vi "servo oscillation_rahul 1.vi"() -> ()   [LabVIEW 2012]
uses:
  <vilib>/Motion/FlexMotion/FunctionsVIs/AxisResourceConfig.llb/Enable Axes (8 axes).flx
  <vilib>/Motion/FlexMotion/FunctionsVIs/Trajectory.llb/Load Acceleration/Deceleration.flx
  <vilib>/Motion/FlexMotion/FunctionsVIs/StartStopMotion.llb/Blend Motion (8 axes).flx
  <vilib>/Motion/FlexMotion/FunctionsVIs/StartStopMotion.llb/Start Motion (8 axes).flx
  <vilib>/Motion/FlexMotion/FunctionsVIs/Trajectory.llb/Check Blend Complete Status (8 axes).flx
  <vilib>/Motion/FlexMotion/FunctionsVIs/Trajectory.llb/Check Move Complete Status (8 axes).flx
  <vilib>/Motion/FlexMotion/FunctionsVIs/StartStopMotion.llb/Stop Motion (8 axes).flx
  <vilib>/Analysis/NI_AALBase.lvlib
panel:
  out "Current Position":dbl(slide) scale=-20000.0..20000.0
  in  "STOP":bool
  in  "samples per cycle":dbl=10.0
  in  "no of cycles":dbl=1.0
  in  "amplitude":dbl=15000.0 format="%0.2f"
  in  "RUN":bool
  in  "Acceleration":dbl=100000.0
  in  "Velocity":dbl=10000.0 min=-20000000.0 max=20000000.0
  in  "Board ID":T1=1 min=1 max=32 step=1
  in  "Axis Cluster":T2
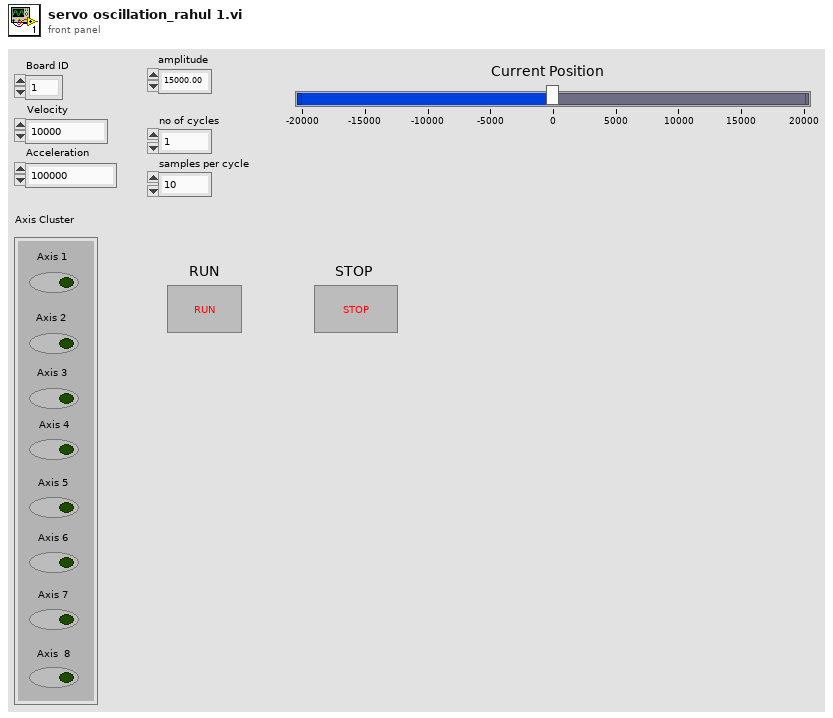
[diagram p1: front panel]
types:
  T1 = typedef "Board Id" = u8
  T2 = cluster{"Axis 1":bool, "Axis 2":bool, "Axis 3":bool, "Axis 4":bool, "Axis 5":bool, "Axis 6":bool, "Axis 7":bool, "Axis  8":bool}
  T3 = enum16{"Absolute Position", "Relative Position", "Velocity", "Relative to Cap Pos", "Modulus Position", "Absolute Contouring", "Relative Contouring"}
  T4 = typedef "Bd Id Out" = u8
  T5 = typedef "Resource Out (Enum).flx" = u16
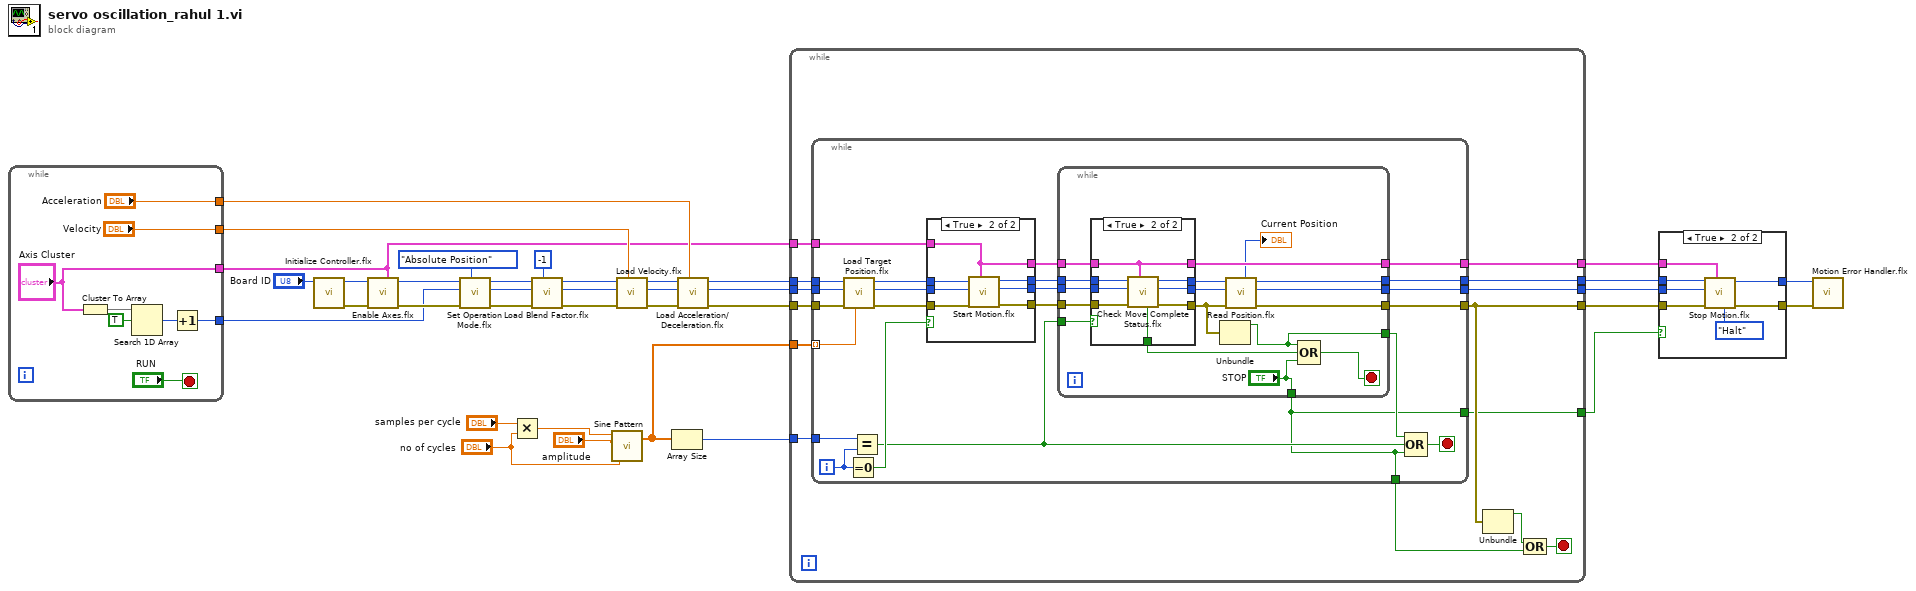
[diagram p0: block diagram]
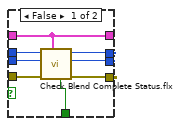
[diagram p2: hidden frame]
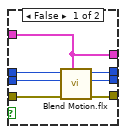
[diagram p3: hidden frame]
diagram:
  n1 = while {
    tunnel: ["Axis Cluster"] -> w14
    tunnel: [w39] -> w20
    tunnel: ["Velocity"] -> w19
    tunnel: ["Acceleration"] -> w18
    stop <- "RUN" stop-if-true
    n2 = Cluster To Array(cluster="Axis Cluster") -> (array=w43:bool[])
    n3 = Search 1D Array(1D array=w43, element=TRUE) -> (index of element=w41:i32)  [unwired: 1 in]
    n4 = Increment(x=w41) -> (x+1=w39:i32)
  }
  n5 = call <vilib>:"Initialize Controller.flx"("Board ID"="Board ID") -> ("error out"=w35:errorcluster, "Bd ID Out"=w36:T4)  [unwired: 7 in]
  n6 = call-poly <vilib>:"Enable Axes.flx"("Axis Bitmap (Disabled)"=w14, "error in (no error)"=w35, "Board ID"=w36) -> ("error out"=w34:errorcluster, "Bd ID Out"=w33:T4)  [unwired: 5 in]
  n7 = call <vilib>:"Set Operation Mode.flx"("Position Mode (Absolute)"=T3."Absolute Position", "error in (no error)"=w34, "Axis or Vector Space"=w20, "Board ID"=w33) -> ("error out"=w26:errorcluster, "Resource Output"=w25:T5, "Bd ID Out"=w27:T4)  [unwired: 2 in]
  n8 = Multiply(x="samples per cycle", y="no of cycles") -> (x*y=w11:dbl)
  n9 = call <vilib>:"Load Blend Factor.flx"("Blend Factor (-1)"=i16 -1, "error in (no error)"=w26, "Axis or Vector Space"=w25, "Board ID"=w27) -> ("error out"=w22:errorcluster, "Resource Output"=w21:T5, "Bd ID Out"=w23:T4)  [unwired: 3 in]
  n10 = call <vilib>:"Sine Pattern.vi"("cycles"="no of cycles", "amplitude"="amplitude", "samples"=w11) -> ("Sinusoidal Pattern"=w9:dbl[])  [unwired: 1 in, 1 out]
  n11 = call <vilib>:"Load Velocity.flx"("Velocity (10000)"=w19, "error in (no error)"=w22, "Axis or Vector Space"=w21, "Board ID"=w23) -> ("error out"=w31:errorcluster, "Resource Output"=w29:T5, "Bd ID Out"=w30:T4)  [unwired: 3 in]
  n12 = Array Size(array=w9) -> (size(s)=w8:i32)
  n13 = call "Load Acceleration/Deceleration.flx"("Acceleration (100000)"=w18, "error in (no error)"=w31, "Axis or Vector Space"=w29, "Board ID"=w30) -> ("error out"=w16:errorcluster, "Resource Output"=w15:T5, "Bd ID Out"=w17:T4)  [unwired: 3 in]
  n14 = while {
    tunnel: w17 -> [w58]
    tunnel: w16 -> [w57]
    tunnel: w15 -> [w56]
    tunnel: w14 -> [w55]
    tunnel: w9 -> [w54]
    tunnel: w8 -> [w53]
    tunnel: [w52] -> w7
    tunnel: [w51] -> w6
    tunnel: [w47] -> w5
    tunnel: [w50] -> w4
    tunnel: [w45] -> w1
    stop <- w49 stop-if-true
    n15 = while {
      tunnel: w58 -> [w81]
      tunnel: w57 -> [w80]
      tunnel: w56 -> [w79]
      tunnel: w55 -> [w74]
      tunnel: [w69] -> w52
      tunnel: [w68] -> w47
      tunnel: [w67] -> w51
      tunnel: w54 -> [w66] mode=indexing
      tunnel: w53 -> [w65]
      tunnel: [w63] -> w50
      tunnel: [w59] -> w48
      tunnel: [w59] -> w45
      i -> [w64]
      stop <- w60 stop-if-true
      n16 = call <vilib>:"Load Target Position.flx"("Target Position (0)"=w66, "error in (no error)"=w80, "Axis"=w79, "Board ID"=w81) -> ("error out"=w76:errorcluster, "Resource Output"=w75:T5, "Bd ID Out"=w77:T4)  [unwired: 3 in]
      n17 = Equal To 0?(x=w64) -> (x = 0?=w78:bool)
      n18 = Equal?(x=w65, y=w64) -> (x = y?=w62:bool)
      n19 = case shown="True" w78 {
        tunnel: w77 -> [w119 w127]
        tunnel: w76 -> [w121 w128]
        tunnel: w75 -> [w118 w126]
        tunnel: w74 -> [w115 w122]
        tunnel: [w117 w125] -> w73
        tunnel: [w120 w124] -> w71
        tunnel: [w116 w123] -> w72
        tunnel: [w115 w122] -> w70
        frame False {
          n20 = call-poly <vilib>:"Blend Motion.flx"("Axis/VS Map (Disabled)"=w115, "error in (no error)"=w121, "Axis or Vector Space"=w118, "Board ID"=w119) -> ("error out"=w120:errorcluster, "Resource Output"=w116:T5, "Bd ID Out"=w117:T4)  [unwired: 2 in]
        }
        frame True {
          n21 = call-poly <vilib>:"Start Motion.flx"("Axis/VS Map (Disabled)"=w122, "error in (no error)"=w128, "Axis or Vector Space"=w126, "Board ID"=w127) -> ("error out"=w124:errorcluster, "Resource Output"=w123:T5, "Bd ID Out"=w125:T4)  [unwired: 2 in]
        }
      }
      n22 = while {
        tunnel: w73 -> [w98]
        tunnel: w72 -> [w96]
        tunnel: w71 -> [w97]
        tunnel: w70 -> [w95]
        tunnel: [w92] -> w69
        tunnel: [w91] -> w68
        tunnel: [w90] -> w67
        tunnel: w62 -> [w89]
        tunnel: [w88] -> w63
        tunnel: [w84] -> w61
        tunnel: ["STOP"] -> w59
        stop <- w85 stop-if-true
        n23 = case shown="True" w89 {
          tunnel: w98 -> [w106 w113]
          tunnel: w97 -> [w104 w114]
          tunnel: w96 -> [w105 w112]
          tunnel: [w103 w111] -> w94
          tunnel: [w102 w109] -> w87
          tunnel: [w101 w110] -> w93
          tunnel: w95 -> [w100 w108]
          tunnel: [w100 w108] -> w88
          tunnel: [w99 w107] -> w86
          frame False {
            n24 = call-poly <vilib>:"Check Blend Complete Status.flx"("Axis/VS Map (Disabled)"=w100, "error in (no error)"=w104, "Axis or Vector Space"=w105, "Board ID"=w106) -> ("error out"=w102:errorcluster, "Resource Output"=w101:T5, "Bd ID Out"=w103:T4, "Blend Complete"=w99:bool)  [unwired: 2 in]
          }
          frame True {
            n25 = call-poly <vilib>:"Check Move Complete Status.flx"("Axis/VS Map (Disabled)"=w108, "error in (no error)"=w114, "Axis or Vector Space"=w112, "Board ID"=w113) -> ("error out"=w109:errorcluster, "Resource Output"=w110:T5, "Bd ID Out"=w111:T4, "Move Complete"=w107:bool)  [unwired: 2 in]
          }
        }
        n26 = Unbundle(w87) -> ("status"=w84:bool)  [unwired: 2 out]
        n27 = call <vilib>:"Read Position.flx"("error in (no error)"=w87, "Axis"=w93, "Board ID"=w94) -> ("error out"=w91:errorcluster, "Resource Output"=w90:T5, "Bd ID Out"=w92:T4, "Position"=→"Current Position":i32)  [unwired: 3 in]
        n28 = Compound Arithmetic op=OR(w84, w86, "STOP") -> (w85:bool)
      }
      n29 = Compound Arithmetic op=OR(w61, w62, w59) -> (w60:bool)
    }
    n30 = Unbundle(w47) -> ("status"=w46:bool)  [unwired: 2 out]
    n31 = Compound Arithmetic op=OR(w46, w48) -> (w49:bool)
  }
  n32 = case shown="True" w1 {
    tunnel: w7 -> [w130 w136]
    tunnel: w6 -> [_ w135]
    tunnel: w5 -> [w129 w137]
    tunnel: w4 -> [_ w134]
    tunnel: [w130 w132] -> w3
    tunnel: [w129 w131] -> w2
    frame False {
    }
    frame True {
      n33 = call-poly <vilib>:"Stop Motion.flx"("Stop Type (Decel)"=enum16{"Decelerate", "Halt", "Kill"}."Halt", "Axis/VS Map (Disabled)"=w134, "error in (no error)"=w137, "Axis or Vector Space"=w135, "Board ID"=w136) -> ("error out"=w131:errorcluster, "Bd ID Out"=w132:T4)  [unwired: 2 in, 1 out]
    }
  }
  n34 = call <vilib>:"Motion Error Handler.flx"("Board ID"=w3, "error in (no error)"=w2) -> ()  [unwired: 9 in, 5 out]
